vi "Get Time from ClockID.vi"(8 "error in (no error)":errorcluster, 9 "Reset Clock T0":bool, 11 "CIFCorePlugin in":refnum<class "CIFCorePlugin.lvclass">) -> (0 "error out":errorcluster, 1 "Clock T0 changed":bool, 2 "ClockID Time (ns)":i64, 3 "CIFCorePlugin out":refnum<class "CIFCorePlugin.lvclass">)   [LabVIEW 2021, in "CIFCorePlugin.lvclass"]
uses:
  CIFCorePlugin.lvclass
  CIFCorePlugin.lvclass/CIFCorePlugin.ctl
  <vilib>/CIF Foundation/CIF Utilities/Time/External Clocks/System Time to External Time.vi
  <vilib>/CIF Foundation/CIF Utilities/Time/System Time/Get System Time.vi
  <vilib>/CIF Foundation/CIF Utilities/Time/SubVIs/Add Error.vi
  <vilib>/CIF Foundation/CIF Utilities/Time/System Time/LabVIEW Time to TAI Time.vi
  <vilib>/CIF Foundation/CIF Utilities/Errors/Append Error Location.vi
  <vilib>/CIF Foundation/CIF Utilities/Time/Time_CIF_U.lvlib
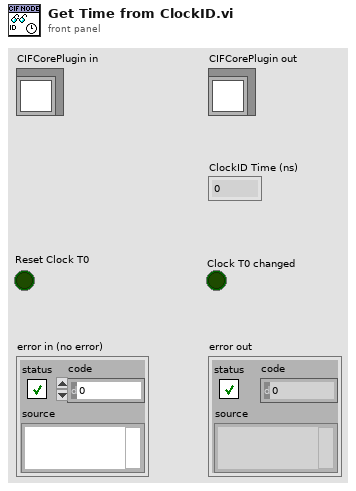
[diagram p1: front panel]
types:
  T1 = typedef "Time_CIF_U.lvlib/Clock Conversion Map.ctl" = map{u8, cluster{"Last Reset":i64, "Offset Pair":T2, "Slope":dbl, "1/Slope":dbl}}
  T2 = typedef "Time_CIF_U.lvlib/Timestamp Pair.ctl" = cluster{"System Time":i64, "External Time":i64}
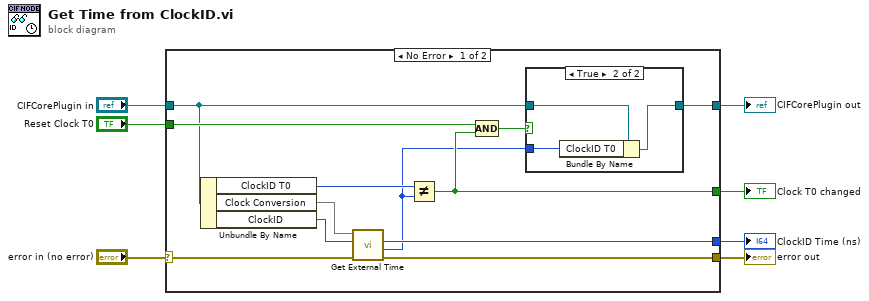
[diagram p0: block diagram]
diagram:
  n1 = case shown="No Error" "error in (no error)" {
    selector: "error in (no error)" -> [w12 w24]
    tunnel: [w11 w24] -> w4
    tunnel: [w15 w25] -> w6
    tunnel: "CIFCorePlugin in" -> [w16 w25]
    tunnel: [w10 _] -> w3
    tunnel: [w18 _] -> w2
    tunnel: "Reset Clock T0" -> [w19 _]
    frame No Error {
      n2 = Unbundle By Name(w16) -> ("ClockID T0"=w9:i64, "Clock Conversion"=w14:T1, "ClockID"=w13:u8)
      n3 = call <vilib>:"Get External Time.vi"("error in (no error)"=w12, "ClockID"=w13, "Clock Convert Map in"=w14) -> ("error out"=w11:errorcluster, "T0"=w8:i64, "Time (ns)"=w10:i64)  [unwired: 5 in, 1 out]
      n4 = Not Equal?(x=w9, y=w8) -> (x != y?=w18:bool)
      n5 = Compound Arithmetic op=AND(w19, w18) -> (w17:bool)
      n6 = case shown="True" w17 {
        tunnel: w8 -> [_ w22]
        tunnel: w16 -> [w20 w23]
        tunnel: [w20 w21] -> w15
        frame False {
        }
        frame True {
          n7 = Bundle By Name(cluster=w23, "ClockID T0"=w22) -> (w21:refnum<class "CIFCorePlugin.lvclass">)
        }
      }
    }
    frame Error {
    }
  }
  "error out" <- w4
  "CIFCorePlugin out" <- w6
  "ClockID Time (ns)" <- w3
  "Clock T0 changed" <- w2
